vi "GetWebpageAndSave.vi"(5 "password":string, 7 "username":string, 8 "Error In":errorcluster, 9 "timeout (ms)":i32=1000, 10 "url":string, 11 "pathIn":path) -> (0 "error out":errorcluster, 3 "pathOut":path)   [LabVIEW 2021]
uses:
  <vilib>/httpClient/ClientHandle.ctl
  38554218-1439-4349-91ca-197dec96393c.vi
  <vilib>/httpClient/LabVIEWHTTPClient.lvlib
panel:
  out "headers":string
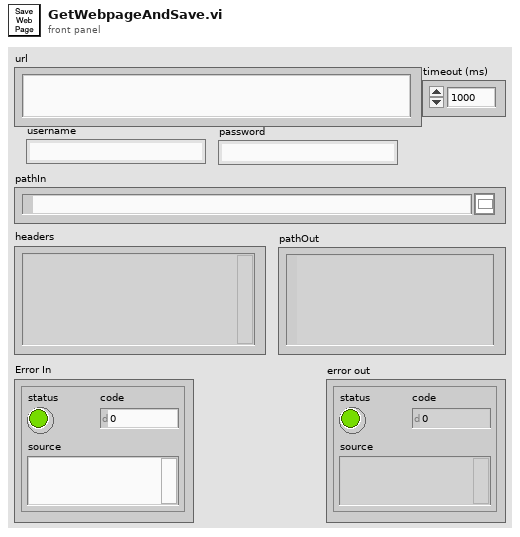
[diagram p1: front panel]
types:
  T1 = typedef "LabVIEWHTTPClient.lvlib/ClientHandle.ctl" = refnum<k1>
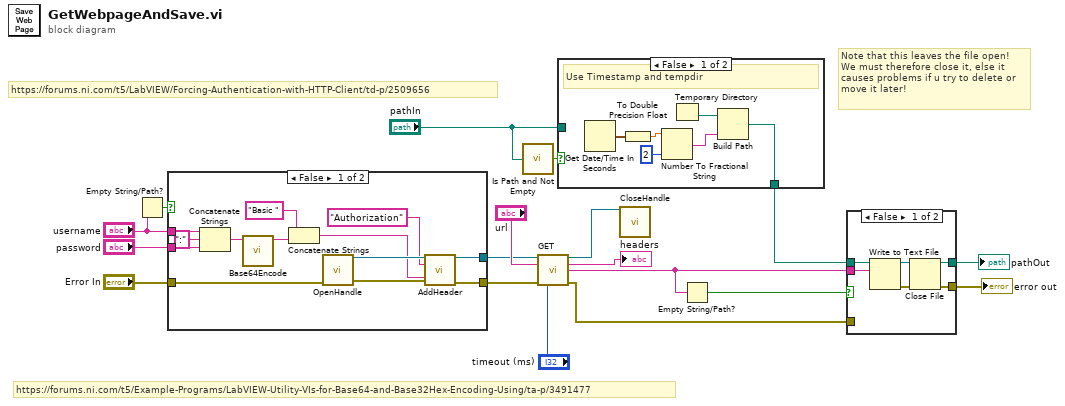
[diagram p0: block diagram]
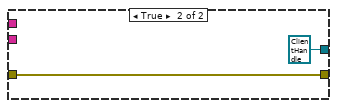
[diagram p3: hidden frame]
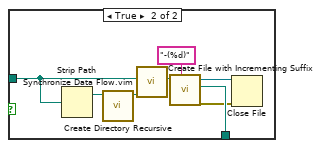
[diagram p4: hidden frame]
diagram:
  # "Note that this leaves the file open!\nWe must therefore close it, else it \ncauses problems if u try to delete or\nmove it later!"
  # "https://forums.ni.com/t5/Example-Programs/LabVIEW-Utility-VIs-for-Base64-and-Base32Hex-Encoding-Using/ta-p/3491477"
  # "https://forums.ni.com/t5/LabVIEW/Forcing-Authentication-with-HTTP-Client/td-p/2509656"
  n1 = Empty String/Path?(string/path="username") -> (empty?=w6:bool)
  n2 = case shown="False" w6 {
    tunnel: [w30 T1 refnum ("client handle out")] -> w11
    tunnel: "Error In" -> [w28 w33]
    tunnel: [w27 w33] -> w8
    tunnel: "username" -> [w25 _]
    tunnel: "password" -> [w24 _]
    frame False {
      n3 = Concatenate Strings(w25, ":" ("string"), w24) -> (w21:string)
      n4 = call "Base64Encode.vi"("String"=w21) -> ("Base64 String"=w22:string)  [unwired: 10 in]
      n5 = Concatenate Strings("Basic ", w22) -> (w20:string)
      n6 = call <vilib>:"OpenHandle.vi"("error in (no error)"=w28) -> ("client handle out"=w31:T1, "error out"=w29:errorcluster)  [unwired: 13 in]
      n7 = call <vilib>:"AddHeader.vi"("client handle"=w31, "header"="Authorization", "value"=w20, "error in (no error)"=w29) -> ("client handle out"=w30:T1, "error out"=w27:errorcluster)  [unwired: 10 in]
    }
    frame True {
    }
  }
  n8 = call <vilib>:"Is Path and Not Empty.vi"("path"="pathIn") -> ("Is Path and Not Empty?"=w16:bool)  [unwired: 4 in]
  n9 = call <vilib>:"GET.vi"("client handle"=w11, "url"="url", "error in (no error)"=w8, "timeout (10000)"="timeout (ms)") -> ("client handle out"=w10:T1, "headers"=→"headers":string, "body"=w3:string, "error out"=w1:errorcluster)  [unwired: 8 in]
  n10 = case shown="False" w16 {
    tunnel: [w39 w47] -> w4
    tunnel: "pathIn" -> [_ w44]
    frame False {
      # "Use Timestamp and tempdir"
      n11 = Get Date/Time In Seconds() -> (seconds since 1Jan1904=w37:timestamp)
      n12 = To Double Precision Float(number=w37) -> (double precision float=w36:dbl)
      n13 = Number To Fractional String(number=w36, precision (6)=i16 2) -> (F-format string=w35:string)  [unwired: 2 in]
      n14 = Temporary Directory() -> (w38:path)
      n15 = Build Path(base path=w38, name or relative path=w35) -> (appended path=w39:path)
    }
    frame True {
      n16 = Strip Path(path=w44) -> (stripped path=w45:path)  [unwired: 1 out]
      n17 = call <vilib>:"Create Directory Recursive.vi"("directory"=w45) -> ("directory copy"=w42:path)  [unwired: 4 in, 2 out]
      n18 = call "Synchronize Data Flow.vim"("input 4"=w42, "input 2"=w44) -> ("output 2"=w43:path)  [unwired: 2 in, 3 out]
      n19 = call <vilib>:"Create File with Incrementing Suffix.vi"("format string (\" (%d)\")"="-(%d)" ("format string (\" (%d)\")"), "file path"=w43) -> ("error out"=w41:errorcluster, "actual path"=w47:path, "refnum out"=w40:refnum<file>)  [unwired: 7 in]
      n20 = Close File(refnum=w40, error in=w41) -> ()  [unwired: 2 out]
    }
  }
  n21 = call <vilib>:"CloseHandle.vi"("client handle"=w10) -> ()  [unwired: 14 in, 1 out]
  n22 = Empty String/Path?(string/path=w3) -> (empty?=w2:bool)
  n23 = case shown="False" w2 {
    tunnel: [w48 w54] -> w18
    tunnel: [w49 w55] -> w14
    tunnel: w4 -> [w53 w55]
    tunnel: w3 -> [w52 _]
    tunnel: w1 -> [_ w54]
    frame False {
      n24 = Write to Text File(file (use dialog)=w53, text=w52) -> (refnum out=w50:refnum<file>, error out=w51:errorcluster)  [unwired: 2 in, 1 out]
      n25 = Close File(refnum=w50, error in=w51) -> (path=w49:path, error out=w48:errorcluster)
    }
    frame True {
    }
  }
  "error out" <- w18
  "pathOut" <- w14
